vi "Client - Main.vi"() -> ()   [LabVIEW 2020]
uses:
  old/controls/States.ctl
  old/controls/Ports to Check.ctl
panel:
  in  "InsightCM Server Address":string="127.0.0.1"
  in  "User Panel":enum32{"User Panel"}(tab)
  in  "stop":bool
  in  "Establish Connection":bool
  in  "Start Test":bool
  in  "View Results":bool
  in  "Log Results":bool
  out "error out":errorcluster
  out "Ports to Check":T1={"TCP Ports"=[82, 482, 5672, 6343, 8002, 49580, 3580, 80, 22, 44516, 52725, 8080], "UDP Ports"=[5353, 44515, 44525]}
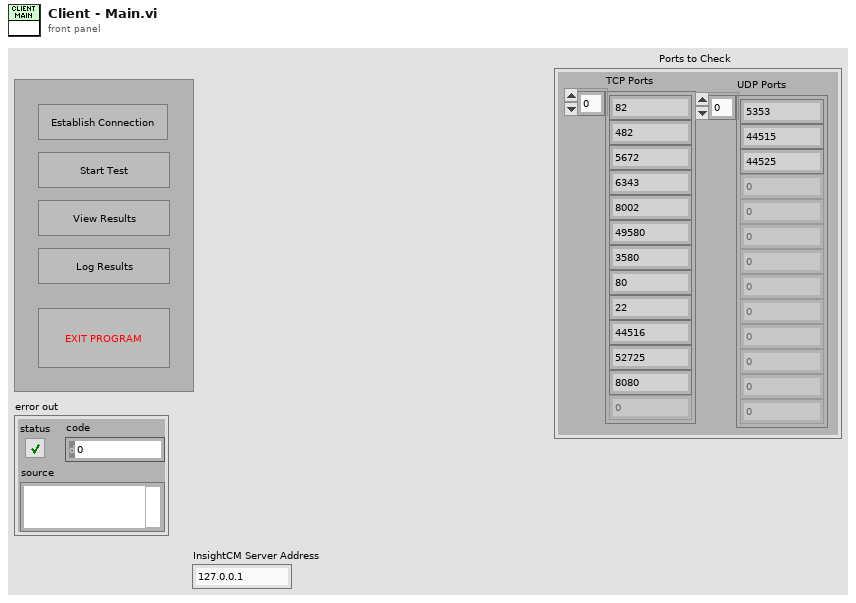
[diagram p1: front panel]
types:
  T1 = typedef "Ports to Check.ctl" = cluster{"TCP Ports":u32[], "UDP Ports":u32[]}
  T2 = typedef "States.ctl" = enum16{"Initialize", "Idle", "Establish Connection", "Start Test", "TCP Tests", "UDP Tests", "Test Complete", "View Results", "Log Results", "Edit Configuration", "Stop"}
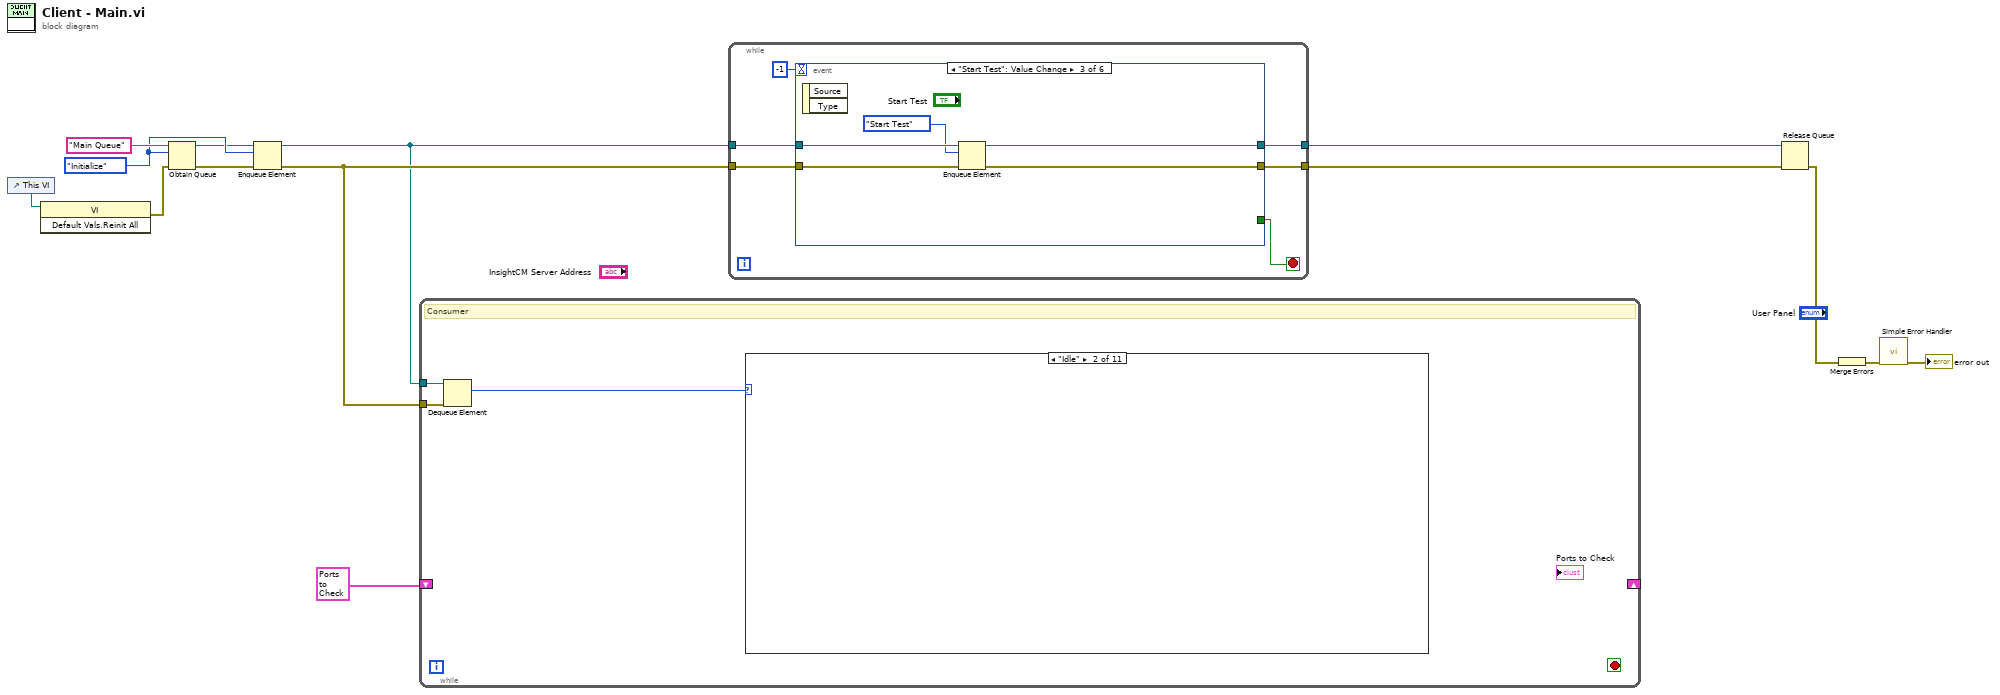
[diagram p0: block diagram]
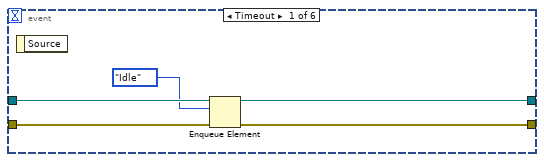
[diagram p2: hidden frame]
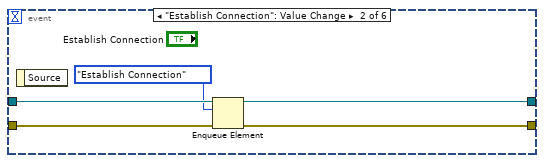
[diagram p3: hidden frame]
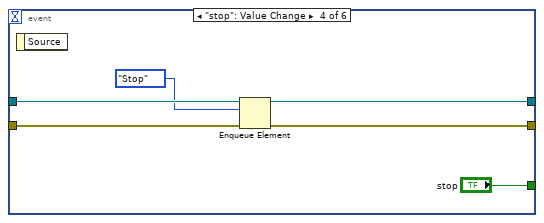
[diagram p4: hidden frame]
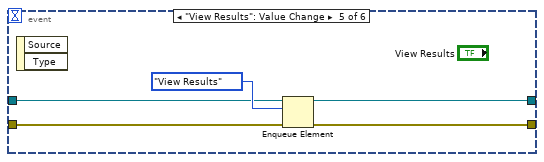
[diagram p5: hidden frame]
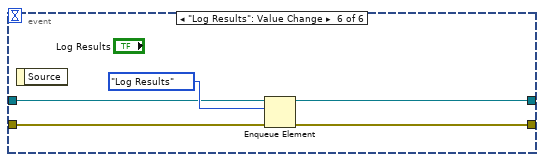
[diagram p6: hidden frame]
diagram:
  w4 = States."Initialize" ("States")
  n1 = control-ref of="This VI"() -> (w7:refnum<vi>)
  n2 = invoke class="VI" method="Default Vals.Reinit All"(reference=w7) -> (error out=w6:errorcluster)  [unwired: 2 in, 2 out]
  n3 = Obtain Queue(name (unnamed)="Main Queue", element data type=w4, error in (no error)=w6) -> (queue out=w2:refnum<queue>, error out=w8:errorcluster)  [unwired: 2 in, 1 out]
  n4 = Enqueue Element(queue=w2, element=w4, error in (no error)=w8) -> (queue out=w3:refnum<queue>, error out=w5:errorcluster)  [unwired: 1 in, 1 out]
  n5 = while {
    tunnel: w3 -> [w17]
    tunnel: w5 -> [w16]
    shift-right: _ -> [_]
    shift-left: T1 {"TCP Ports"=[82, 482, 5672, 6343, 8002, 49580, 3580, 80, 22, 44516, 52725, 8080], "UDP Ports"=[5353, 44515, 44525]} ("Ports to Check") -> [_]
    stop <- _ stop-if-true
    # "Consumer"
    n6 = Dequeue Element(queue=w17, error in (no error)=w16) -> (element=w15:T2)  [unwired: 1 in, 3 out]
    n7 = case shown="\"Idle\"" w15 {
      frame "Initialize", Default {
      }
      frame "Idle" {
      }
      frame "Establish Connection" {
      }
      frame "Start Test" {
      }
      frame "TCP Tests" {
      }
      frame "UDP Tests" {
      }
      frame "Test Complete" {
      }
      frame "View Results" {
      }
      frame "Log Results" {
      }
      frame "Edit Configuration" {
      }
      frame "Stop" {
      }
    }
  }
  n8 = while {
    tunnel: w3 -> [w23]
    tunnel: [w22] -> w13
    tunnel: w5 -> [w20]
    tunnel: [w19] -> w10
    stop <- w21 stop-if-true
    n9 = event shown="[2] \"Start Test\": Value Change" {
      selector: _ -> [_ _ _ _ _ _]
      dyn-events: _ -> [_ _ _ _ _ _]
      timeout: -1 -> [_ _ _ _ _ _]
      tunnel: w23 -> [w28 w33 w38 w43 w48 w53]
      tunnel: [w27 w31 w36 w42 w47 w52] -> w22
      tunnel: [_ _ _ "stop" _ _] -> w21
      tunnel: w20 -> [w26 w30 w35 w40 w46 w51]
      tunnel: [w25 w29 w34 w39 w45 w50] -> w19
      event Timeout {
        n10 = event-data() -> ()  [unwired: 1 in, 1 out]
        n11 = Enqueue Element(queue=w28, element=States."Idle" ("States"), error in (no error)=w26) -> (queue out=w27:refnum<queue>, error out=w25:errorcluster)  [unwired: 1 in, 1 out]
      }
      event "Establish Connection": Value Change {
        n12 = event-data() -> ()  [unwired: 1 in, 1 out]
        n13 = Enqueue Element(queue=w33, element=States."Establish Connection" ("States"), error in (no error)=w30) -> (queue out=w31:refnum<queue>, error out=w29:errorcluster)  [unwired: 1 in, 1 out]
      }
      event "Start Test": Value Change {
        n14 = event-data() -> ()  [unwired: 1 in, 2 out]
        n15 = Enqueue Element(queue=w38, element=States."Start Test" ("States"), error in (no error)=w35) -> (queue out=w36:refnum<queue>, error out=w34:errorcluster)  [unwired: 1 in, 1 out]
      }
      event "stop": Value Change {
        n16 = event-data() -> ()  [unwired: 1 in, 1 out]
        n17 = Enqueue Element(queue=w43, element=States."Stop" ("States"), error in (no error)=w40) -> (queue out=w42:refnum<queue>, error out=w39:errorcluster)  [unwired: 1 in, 1 out]
      }
      event "View Results": Value Change {
        n18 = event-data() -> ()  [unwired: 1 in, 2 out]
        n19 = Enqueue Element(queue=w48, element=States."View Results" ("States"), error in (no error)=w46) -> (queue out=w47:refnum<queue>, error out=w45:errorcluster)  [unwired: 1 in, 1 out]
      }
      event "Log Results": Value Change {
        n20 = event-data() -> ()  [unwired: 1 in, 1 out]
        n21 = Enqueue Element(queue=w53, element=States."Log Results" ("States"), error in (no error)=w51) -> (queue out=w52:refnum<queue>, error out=w50:errorcluster)  [unwired: 1 in, 1 out]
      }
    }
  }
  n22 = Release Queue(queue=w13, error in (no error)=w10) -> (error out=w9:errorcluster)  [unwired: 1 in, 2 out]
  n23 = Merge Errors(w9) -> (w11:errorcluster)
  n24 = call <vilib>:"Simple Error Handler.vi"("error in (no error)"=w11) -> ("error out"=→"error out":errorcluster)  [unwired: 4 in, 4 out]
